vi "多个线圈写入.vi"(8 "Error in":errorcluster caption="Error in (no error)", 9 "values":bool[](array[boolean]), 10 "starting address":u16, 11 "Slave ID":u8=10) -> (0 "error out":errorcluster)   [LabVIEW 2016, in "质控单元.lvlib"]
uses:
  <vilib>/Plasmionique/MB Master/MB_Master/MB_Master.lvclass
  <vilib>/Plasmionique/MB Master/MB Master.lvlib
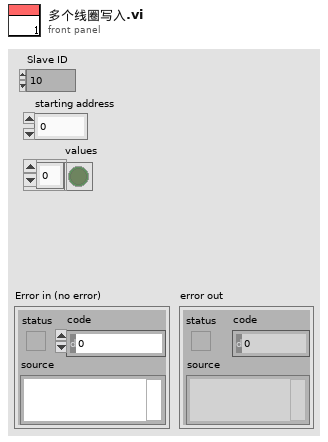
[diagram p1: front panel]
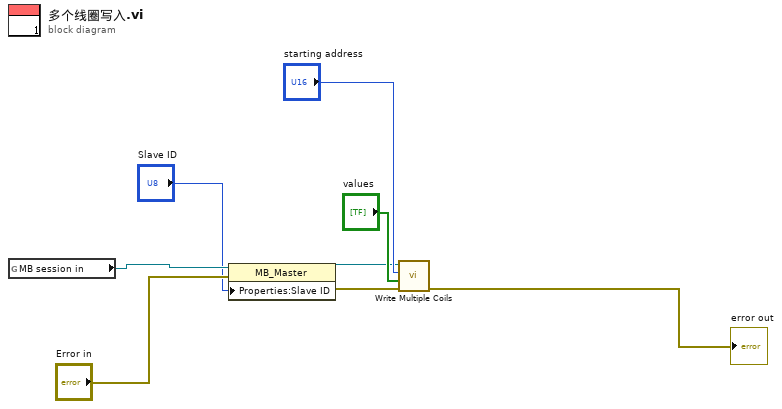
[diagram p0: block diagram]
diagram:
  n1 = global read "断电保存全局.vi" "MB session in"() -> (w6:refnum<class "MB_Master.lvclass">)
  n2 = property class="MB_Master"(reference=w6, error in="Error in", "Properties:Slave ID"="Slave ID") -> (reference out=w5:refnum<class "MB_Master.lvclass">, error out=w4:errorcluster)
  n3 = call <vilib>:"Write Multiple Coils.vi"("error in (no error)"=w4, "values"="values", "starting address"="starting address", "MB session in"=w5) -> ("error out"=→"error out":errorcluster)  [unwired: 6 in, 1 out]
